vi "Day 2-1.vi"() -> ()   [LabVIEW 2022 SP3]
uses:
  <vilib>/Utility/error.llb/Trim Whitespace One-Sided.vi
panel:
  out "Part 2":i32
  out "Part 1":i32
  in  "Max":cluster{"red":i32, "green":i32, "blue":i32}={"red"=12, "green"=13, "blue"=14}
  in  "String":string="Game 1: 4 green, 7 blue; 2 blue, 4 red; 5 blue, 2 green, 2 red; 1 green, 3 red, 9 blue; 3 green, 9 blue; 7 green, 2 blue, 2 red\nGame 2: 1 blue, 2 red; 1 green, 2 blue, 1 red; 1 red, 5 green; 3 red, 2 blue, 8 green; 3 blue, 2 red, 4 green; 2 blue, 4 green, 3 red\nGame 3: 7 red, 7 blue, 9 green; 15 green, 4 red, 8 blue; 3 green, 12 blue, 6 red\nGame 4: 4 blue, 11 green, 6 red; 4 green, 2 red; 12 red, 1 blue, 3 green\nGame 5: 10 green, 4 blue, 9 red; 3 green, 15 blue, 11 red; 15 blue, 1 green, 2 red; 8 red, 8 blue, 5 green\nGame 6: 5 green, 19 red; 6 green, 13 red, 2 blue; 2 blue, 16 red, 4 green; 13 red, 9 blue, 5 green\nGame 7: 1 blue, 6 red, 6 green; 7 blue, 4 red; 6 green, 1 red, 11 blue; 3 green, 4 blue, 4 red; 6 green, 13 blue, 11 red\nGame 8: 8 green, 2 blue; 20 green, 1 red; 1 blue, 6 red, 6 green; 9 green\nGame 9: 5 red; 4 green, 3 red, 1 blue; 1 blue; 6 red, 1 blue, 9 green\nGame 10: 2 green, 3 red; 18 blue, 20 green, 9 red; 7 red, 9 blue, 17 green\nGame 11: 15 green, 7 blue, 9 red; 7 blue, 10 green, 7 red; 5 red, 3 blue, 10 green; 5 blue, 12 green; 14 green, 8 blue, 5 red; 7 blue, 2 red, 5 green\nGame 12: 3 green, 1 red, 8 blue; 9 blue, 3 red, 3 green; 4 blue, 1 green; 2 red, 3 green, 1 blue; 4 red, 7 blue, 3 green\nGame 13: 14 green, 1 red; 4 green; 2 green, 1 blue; 14 green; 13 green, 1 red, 1 blue; 1 blue, 1 red, 5 green\nGame 14: 1 blue, 6 red, 13 green; 5 red, 10 blue, 3 green; 19 green, 1 red, 14 blue; 4 red, 17 green, 9 blue; 12 green, 10 blue, 7 red\nGame 15: 10 red, 2 blue, 18 green; 17 green, 3 blue, 7 red; 18 blue, 8 red, 12 green; 6 blue, 6 green, 12 red\nGame 16: 14 blue, 5 green, 12 red; 7 green, 3 red, 9 blue; 4 green, 1 red, 8 blue; 9 red, 19 green, 12 blue; 12 blue, 7 red, 6 green; 5 blue, 3 green, 6 red\nGame 17: 1 green, 1 blue, 15 red; 1 blue, 3 green, 12 red; 9 blue, 2 green, 10 red\nGame 18: 12 red, 7 green, 7 blue; 3 blue, 8 red, 1 green; 2 green, 17 red\nGame 19: 1 red, 7 blue, 17 green; 11 red, 15 blue; 11 blue, 18 green; 6 blue, 14 green, 14 red; 16 blue, 8 red, 8 green; 17 green, 9 red, 1 blue\nGame 20: 11 green; 1 blue, 4 green, 7 red; 7 green; 3 red, 1 blue, 6 green\nGame 21: 18 blue, 6 green, 10 red; 12 blue; 9 blue, 2 green, 9 red; 9 red, 20 blue, 1 green; 8 blue, 6 red; 19 blue, 1 green, 4 red\nGame 22: 4 blue, 16 red, 3 green; 7 blue, 3 green, 12 red; 10 red, 7 green, 10 blue; 7 red, 11 blue, 4 green; 3 blue, 1 green, 16 red\nGame 23: 5 green, 8 red, 1 blue; 2 red, 5 blue, 3 green; 2 green, 17 blue, 4 red; 2 blue, 2 red; 7 red, 1 green, 14 blue; 4 red, 8 blue\nGame 24: 1 blue, 3 green, 1 red; 3 blue, 11 green, 15 red; 3 blue, 2 red, 12 green; 9 green, 6 red, 2 blue; 15 green, 12 red, 3 blue; 13 green, 1 blue, 13 red\nGame 25: 6 blue, 5 red, 10 green; 9 red, 3 blue, 3 green; 6 blue, 11 red, 15 green; 7 green, 10 red, 4 blue; 2 red, 20 blue, 11 green\nGame 26: 3 blue, 5 red, 10 green; 7 green, 6 red; 7 green, 1 red, 3 blue; 10 green, 4 red, 3 blue; 4 red, 7 green, 3 blue; 8 green, 4 red\nGame 27: 16 green, 6 blue, 4 red; 3 red, 6 blue, 7 green; 10 green; 6 green, 1 red\nGame 28: 5 green, 5 red, 2 blue; 1 blue, 9 red, 6 green; 2 blue, 3 red; 1 blue, 1 green, 5 red; 4 green, 3 red; 9 green, 1 blue, 14 red\nGame 29: 1 red, 2 green, 13 blue; 1 green, 2 red, 9 blue; 12 red; 3 blue, 5 red\nGame 30: 8 blue, 3 red, 9 green; 10 green, 9 blue; 9 green, 12 blue; 3 blue, 2 red, 4 green; 8 blue, 9 green; 1 red, 12 blue, 6 green\nGame 31: 8 red, 16 blue; 2 red, 1 green, 1 blue; 5 red, 8 blue, 1 green\nGame 32: 3 green, 5 blue, 8 red; 10 blue, 1 red, 3 green; 9 green, 3 blue, 2 red; 2 blue, 1 red, 14 green; 3 blue, 10 red, 16 green\nGame 33: 1 red, 3 green, 2 blue; 15 blue, 1 green; 1 green, 1 red, 10 blue\nGame 34: 4 green, 7 blue; 2 blue, 12 green; 6 red, 14 green, 7 blue\nGame 35: 9 blue, 1 green; 2 green, 6 blue, 11 red; 1 green, 10 red, 1 blue\nGame 36: 5 blue, 1 green, 2 red; 11 blue, 3 green, 5 red; 2 green, 14 blue, 2 red; 3 green, 5 blue, 5 red; 13 blue, 2 green, 5 red; 3 green\nGame 37: 4 blue, 2 red, 8 green; 1 blue, 9 green, 4 red; 1 red, 4 green, 1 blue; 16 green, 3 blue, 4 red\nGame 38: 9 blue, 9 green; 1 green, 3 blue; 8 blue, 6 red, 5 green; 1 green, 9 red, 1 blue\nGame 39: 1 red, 17 green; 1 blue, 7 green, 7 red; 6 red, 4 blue\nGame 40: 1 blue, 2 red; 10 blue, 4 green, 2 red; 1 green, 11 blue, 3 red; 4 blue, 2 green; 3 blue, 4 red\nGame 41: 7 red, 4 blue, 4 green; 10 red, 11 blue, 1 green; 6 red, 6 blue, 4 green; 13 blue, 3 red, 7 green; 9 green, 12 blue, 14 red; 9 blue, 12 red, 10 green\nGame 42: 3 blue, 1 red, 11 green; 4 blue, 9 green, 8 red; 3 red, 5 blue, 1 green\nGame 43: 2 green, 17 blue, 9 red; 16 red, 12 blue, 2 green; 12 red, 12 blue, 7 green; 17 red, 16 blue, 7 green\nGame 44: 2 red, 3 green, 5 blue; 5 red, 5 blue, 7 green; 2 red, 5 blue, 5 green; 6 red, 5 blue, 2 green\nGame 45: 9 green, 1 blue; 1 red, 5 green, 2 blue; 2 blue, 4 green, 9 red; 13 green, 7 red, 1 blue; 3 blue, 4 green\nGame 46: 5 green, 7 red; 8 green, 5 blue, 1 red; 1 blue, 7 red, 17 green\nGame 47: 1 green, 17 blue; 9 blue, 1 green; 1 blue, 1 red\nGame 48: 1 red, 6 green, 7 blue; 9 green, 1 red, 2 blue; 10 blue, 6 green, 1 red; 1 red, 4 green, 9 blue; 6 blue, 3 green, 1 red\nGame 49: 1 red, 1 blue, 16 green; 3 red, 1 green; 16 green; 2 blue, 8 red, 19 green; 20 green, 9 red; 8 green, 6 red\nGame 50: 1 green, 2 blue; 2 red, 3 blue; 4 red, 2 blue; 1 green; 3 blue; 3 blue, 2 green, 1 red\nGame 51: 6 blue, 5 green; 6 red, 5 green; 6 green, 6 blue, 16 red; 10 red, 10 green, 1 blue\nGame 52: 4 red, 5 green, 1 blue; 15 green, 1 blue; 8 green, 5 blue, 5 red; 4 blue, 11 green, 1 red\nGame 53: 5 green, 3 blue, 5 red; 2 red, 4 blue, 1 green; 1 red, 2 green; 11 red\nGame 54: 7 green, 16 blue, 5 red; 5 green; 10 blue, 6 green, 5 red; 3 green\nGame 55: 3 green; 16 green, 1 blue; 13 green, 19 blue, 1 red; 13 green, 18 blue\nGame 56: 9 green; 3 blue, 1 red, 10 green; 1 red, 4 blue, 9 green\nGame 57: 14 blue, 2 red, 3 green; 1 red, 8 blue, 7 green; 1 green, 3 red, 15 blue; 5 green, 12 blue; 4 green, 15 blue\nGame 58: 9 red, 5 green; 10 green, 11 red, 1 blue; 12 green, 17 red, 1 blue; 1 blue, 1 green, 17 red; 14 red, 1 blue, 16 green\nGame 59: 2 red, 12 blue, 10 green; 6 green, 1 red, 14 blue; 14 blue, 9 green, 2 red; 12 green, 14 blue, 2 red\nGame 60: 5 blue, 8 green; 1 red, 6 green, 7 blue; 1 blue\nGame 61: 5 red, 2 blue, 5 green; 2 blue, 11 green; 1 blue, 2 red, 14 green; 3 green; 4 red, 13 green; 2 blue, 6 green, 1 red\nGame 62: 1 red, 1 blue, 2 green; 3 red, 1 blue, 2 green; 1 blue, 10 red; 6 red, 1 blue\nGame 63: 7 red, 6 blue, 4 green; 2 blue, 5 green, 8 red; 5 blue, 4 green, 10 red; 4 blue, 7 red, 10 green; 5 blue, 10 green, 8 red; 4 blue, 10 green, 3 red\nGame 64: 6 red, 7 green, 15 blue; 8 blue, 16 green, 3 red; 11 green, 12 blue; 4 red, 17 blue, 8 green\nGame 65: 2 blue, 7 green; 2 red, 8 blue; 2 green, 1 red, 5 blue; 1 green, 2 blue; 19 green, 7 blue; 2 red, 3 blue, 14 green\nGame 66: 15 green, 7 blue; 9 blue, 3 green, 16 red; 1 red, 1 blue, 16 green; 18 red, 8 blue, 11 green\nGame 67: 1 blue, 1 green, 2 red; 5 green, 8 red, 2 blue; 7 red, 1 blue\nGame 68: 3 blue, 10 red; 13 red, 1 green; 5 blue, 5 red; 2 blue, 1 green, 16 red; 16 red, 3 blue\nGame 69: 7 red, 1 blue, 3 green; 14 green, 2 blue; 3 green, 2 blue; 4 red, 1 green, 1 blue; 10 red, 14 green, 2 blue\nGame 70: 10 green, 12 red; 5 red, 7 green; 1 blue, 6 red, 11 green\nGame 71: 16 green, 13 red, 10 blue; 7 red, 7 blue, 15 green; 17 green, 13 red, 1 blue; 5 blue, 8 green, 11 red; 7 red, 1 blue, 15 green; 15 green, 4 blue, 2 red\nGame 72: 3 blue, 3 red; 2 blue, 3 red, 1 green; 1 red, 1 blue, 3 green; 1 green, 2 blue, 3 red; 3 blue, 1 green, 1 red; 1 blue, 4 red\nGame 73: 10 blue, 11 red, 5 green; 6 green, 9 blue, 4 red; 10 red, 5 green, 9 blue\nGame 74: 6 green, 17 blue; 1 red, 1 blue, 11 green; 2 blue, 1 red, 3 green\nGame 75: 11 red, 11 green, 3 blue; 11 red, 1 blue, 6 green; 4 green, 3 blue, 8 red\nGame 76: 3 green, 3 blue, 12 red; 3 blue, 15 green, 3 red; 4 red, 15 green, 2 blue\nGame 77: 13 blue, 11 red, 1 green; 3 red, 12 green, 12 blue; 7 red, 15 green, 4 blue; 5 red, 2 green, 3 blue\nGame 78: 4 red, 8 blue, 2 green; 7 blue, 3 green, 7 red; 3 green, 13 blue; 3 red, 4 green\nGame 79: 7 blue, 13 red, 8 green; 7 green, 15 red, 9 blue; 2 green, 8 red, 10 blue; 13 blue, 20 red, 7 green; 11 red, 2 green, 14 blue\nGame 80: 12 red; 2 blue, 15 red, 3 green; 1 blue, 1 green, 2 red; 1 green; 1 green, 3 blue, 13 red; 1 green, 2 blue, 1 red\nGame 81: 11 blue; 6 blue, 8 green, 4 red; 7 blue, 1 red, 1 green\nGame 82: 9 blue, 1 red; 3 blue, 1 red, 3 green; 8 blue, 8 green, 2 red; 5 blue\nGame 83: 7 blue, 13 red; 4 blue, 2 green, 3 red; 15 blue, 9 red, 1 green; 14 red, 1 green, 12 blue\nGame 84: 8 blue, 1 green, 20 red; 9 green, 20 red, 18 blue; 16 red, 15 blue, 5 green; 15 red, 10 green, 16 blue; 11 green, 14 red, 12 blue\nGame 85: 1 red, 2 blue, 9 green; 13 green, 3 blue, 5 red; 1 green, 1 red, 3 blue; 8 green, 2 blue, 1 red\nGame 86: 10 red, 6 blue, 11 green; 1 red, 11 green; 7 blue, 6 red, 11 green\nGame 87: 14 red, 4 blue, 4 green; 14 red, 4 blue, 7 green; 12 red, 11 green, 5 blue; 5 blue, 12 red\nGame 88: 3 green, 4 blue, 11 red; 3 green, 4 blue, 3 red; 10 red, 3 green; 3 blue, 2 red, 2 green\nGame 89: 4 blue, 2 red, 3 green; 3 green, 7 red, 13 blue; 1 green, 6 blue\nGame 90: 7 red; 5 blue, 11 red, 8 green; 8 red, 3 green, 2 blue\nGame 91: 2 blue; 4 red; 2 blue, 4 green; 3 green, 1 blue, 1 red\nGame 92: 7 blue, 10 green; 9 green, 9 blue, 7 red; 6 green; 12 red, 1 blue, 4 green; 5 red, 1 green, 13 blue\nGame 93: 7 green, 6 red, 1 blue; 3 red, 6 green, 8 blue; 1 blue, 6 green; 6 red, 15 blue, 4 green; 10 blue, 2 green, 6 red; 3 green, 5 red, 6 blue\nGame 94: 5 red, 1 green, 15 blue; 1 blue, 6 red; 2 red, 6 blue, 2 green\nGame 95: 9 blue, 4 red, 17 green; 15 green, 9 red, 10 blue; 1 blue, 13 green, 12 red\nGame 96: 1 blue, 12 green, 1 red; 3 blue, 1 green, 5 red; 2 blue, 8 red, 10 green\nGame 97: 18 blue, 7 red, 11 green; 6 red, 3 blue, 14 green; 1 red, 13 blue, 4 green\nGame 98: 5 blue, 2 green, 8 red; 12 red; 13 red, 4 blue, 4 green; 7 red, 11 blue; 10 blue, 2 green, 2 red; 6 red, 12 blue\nGame 99: 4 green, 2 blue, 4 red; 9 blue, 11 red, 1 green; 5 green\nGame 100: 2 blue, 12 green; 6 green, 1 red, 12 blue; 1 green, 5 blue, 1 red; 1 red, 12 green, 6 blue; 16 blue, 3 green"
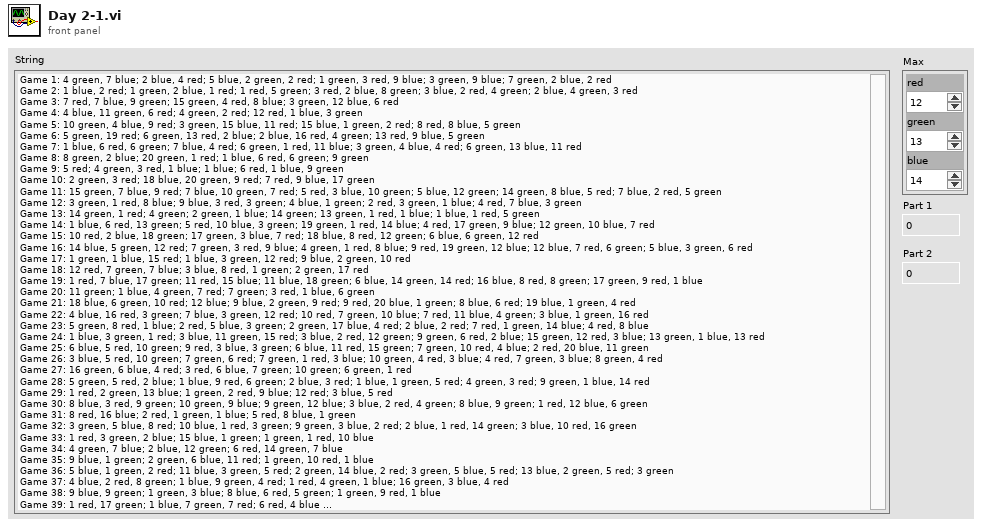
[diagram p1: front panel]
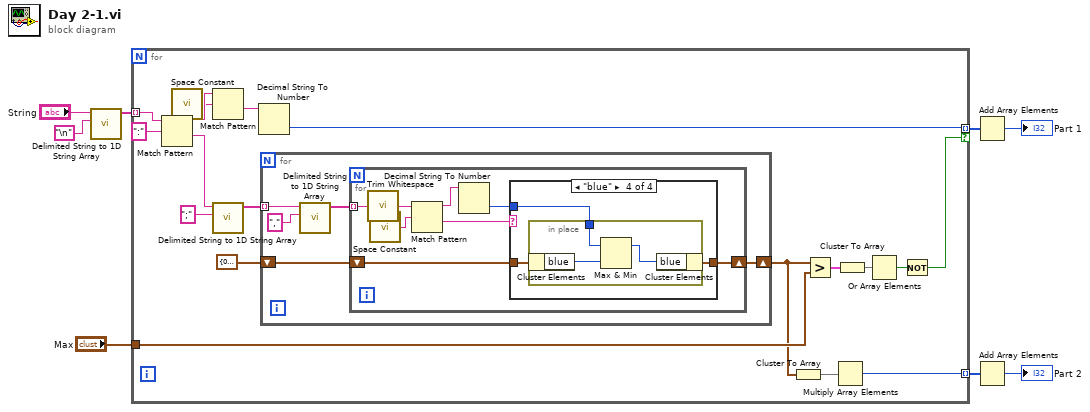
[diagram p0: block diagram]
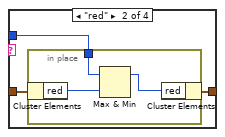
[diagram p3: hidden frame]
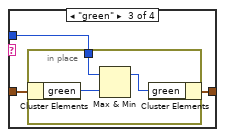
[diagram p4: hidden frame]
diagram:
  n1 = call <vilib>:"Delimited String to 1D String Array.vi"("delimiter"="\n", "delimited string"="String") -> ("string array"=w6:string[])  [unwired: 9 in]
  n2 = for {
    tunnel: w6 -> [w14] mode=indexing
    tunnel: [w20] -> w4 mode=indexing if=w12
    tunnel: "Max" -> [w17]
    tunnel: [w9] -> w2 mode=indexing
    n3 = Match Pattern(string=w14, regular expression=":") -> (before substring=w23:string, after substring=w25:string)  [unwired: 1 in, 2 out]
    n4 = call <vilib>:"Space Constant.vi"() -> ("String"=w22:string)
    n5 = Match Pattern(string=w23, regular expression=w22) -> (after substring=w21:string)  [unwired: 1 in, 3 out]
    n6 = call <vilib>:"Delimited String to 1D String Array.vi"("delimiter"=";", "delimited string"=w25) -> ("string array"=w18:string[])  [unwired: 9 in]
    n7 = Decimal String To Number(string=w21) -> (number=w20:i32)  [unwired: 2 in, 1 out]
    n8 = for {
      shift-right: [w27] -> w11
      shift-left: cluster{"red":i32, "green":i32, "blue":i32} {"red"=0, "green"=0, "blue"=0} -> [w29]
      tunnel: w18 -> [w31] mode=indexing
      n9 = call <vilib>:"Delimited String to 1D String Array.vi"("delimiter"=",", "delimited string"=w31) -> ("string array"=w28:string[])  [unwired: 9 in]
      n10 = for {
        shift-right: [w33] -> w27
        shift-left: w29 -> [w32]
        tunnel: w28 -> [w39] mode=indexing
        n11 = call <vilib>:"Trim Whitespace.vi"("string"=w39) -> ("trimmed string"=w38:string)  [unwired: 1 in]
        n12 = call <vilib>:"Space Constant.vi"() -> ("String"=w37:string)
        n13 = Match Pattern(string=w38, regular expression=w37) -> (before substring=w36:string, after substring=w35:string)  [unwired: 1 in, 2 out]
        n14 = Decimal String To Number(string=w36) -> (number=w34:i32)  [unwired: 2 in, 1 out]
        n15 = case shown="\"blue\"" w35 {
          tunnel: w34 -> [_ w42 w48 w54]
          tunnel: [w40 w41 w47 w53] -> w33
          tunnel: w32 -> [w40 w43 w49 w55]
          frame Default {
          }
          frame "red" {
            n16 = in-place {
              in-place-border: w42 -> [w45]
              n17 = in-place-cluster #1(w43) -> ("red"=w46:i32)
              n18 = Max & Min(x=w45, y=w46) -> (max(x,y)=w44:i32)  [unwired: 1 out]
              n19 = in-place-cluster #1("red"=w44) -> (w41:cluster{"red":i32, "green":i32, "blue":i32})
            }
          }
          frame "green" {
            n20 = in-place {
              in-place-border: w48 -> [w51]
              n21 = in-place-cluster #2(w49) -> ("green"=w52:i32)
              n22 = Max & Min(x=w51, y=w52) -> (max(x,y)=w50:i32)  [unwired: 1 out]
              n23 = in-place-cluster #2("green"=w50) -> (w47:cluster{"red":i32, "green":i32, "blue":i32})
            }
          }
          frame "blue" {
            n24 = in-place {
              in-place-border: w54 -> [w57]
              n25 = in-place-cluster #3(w55) -> ("blue"=w58:i32)
              n26 = Max & Min(x=w57, y=w58) -> (max(x,y)=w56:i32)  [unwired: 1 out]
              n27 = in-place-cluster #3("blue"=w56) -> (w53:cluster{"red":i32, "green":i32, "blue":i32})
            }
          }
        }
      }
    }
    n28 = Cluster To Array(cluster=w11) -> (array=w10:i32[])
    n29 = Greater?(x=w11, y=w17) -> (0:w16:cluster{"red":bool, "green":bool, "blue":bool})
    n30 = Multiply Array Elements(1:w10) -> (0:w9:i32)
    n31 = Cluster To Array(cluster=w16) -> (array=w15:bool[])
    n32 = Or Array Elements(Boolean array=w15) -> (logical OR=w13:bool)
    n33 = Not(x=w13) -> (.not. x?=w12:bool)
  }
  n34 = Add Array Elements(numeric array=w4) -> (sum=→"Part 1":i32)
  n35 = Add Array Elements(numeric array=w2) -> (sum=→"Part 2":i32)
